vi "RD_I2C_CT_ADC.vi"(1 "READ address":u8 format="%x", 2 "NUM_BYTES":u8 format="%x", 3 "DEV address 2":u16 format="%x") -> (0 "DATA 7":u32 format="%x")   [LabVIEW 2016]
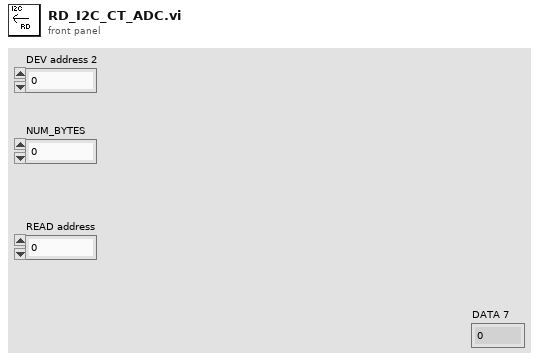
[diagram p1: front panel]
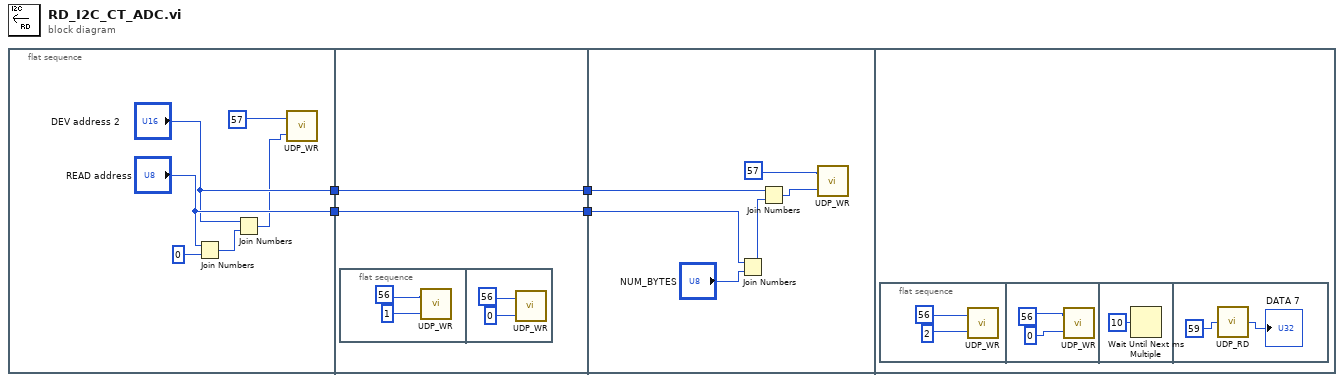
[diagram p0: block diagram]
diagram:
  n1 = flat-sequence {
    tunnel: ["READ address"] -> w4
    tunnel: ["DEV address 2"] -> w2
    tunnel: w4 -> [w12]
    tunnel: [w12] -> w3
    tunnel: w2 -> [w11]
    tunnel: [w11] -> w1
    tunnel: w3 -> [w21]
    tunnel: w1 -> [w19]
    frame #0 {
      n2 = Join Numbers(hi="READ address", lo=u8 0) -> ((hi.lo)=w9:u16)
      n3 = Join Numbers(hi="DEV address 2", lo=w9) -> ((hi.lo)=w5:u32)
      n4 = call "UDP_WR.vi"("DATA"=w5, "ADDRESS"=u16 57) -> ()  [unwired: 1 out]
    }
    frame #1 {
      n5 = flat-sequence {
        frame #0 {
          n6 = call "UDP_WR.vi"("DATA"=u32 1, "ADDRESS"=u16 56) -> ()  [unwired: 1 out]
        }
        frame #1 {
          n7 = call "UDP_WR.vi"("DATA"=u32 0, "ADDRESS"=u16 56) -> ()  [unwired: 1 out]
        }
      }
    }
    frame #2 {
      n8 = Join Numbers(hi=w21, lo="NUM_BYTES") -> ((hi.lo)=w20:u16)
      n9 = Join Numbers(hi=w19, lo=w20) -> ((hi.lo)=w17:u32)
      n10 = call "UDP_WR.vi"("DATA"=w17, "ADDRESS"=u16 57) -> ()  [unwired: 1 out]
    }
    frame #3 {
      n11 = flat-sequence {
        frame #0 {
          n12 = call "UDP_WR.vi"("DATA"=u32 2, "ADDRESS"=u16 56) -> ()  [unwired: 1 out]
        }
        frame #1 {
          n13 = call "UDP_WR.vi"("DATA"=u32 0, "ADDRESS"=u16 56) -> ()  [unwired: 1 out]
        }
        frame #2 {
          n14 = Wait Until Next ms Multiple(millisecond multiple=u32 10) -> ()  [unwired: 1 out]
        }
        frame #3 {
          n15 = call "UDP_RD.vi"("ADDRESS 2"=i16 59) -> ("DATA 2"=→"DATA 7":u32)
        }
      }
    }
  }
